vi "Accelerometer Angle.vi"(10 "angle LPF":dbl=0.02 format="%#_13g", 11 "Values":dbl[](array[numeric])) -> (3 "Numeric":dbl)   [LabVIEW 2014]
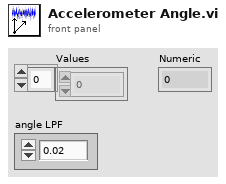
[diagram p1: front panel]
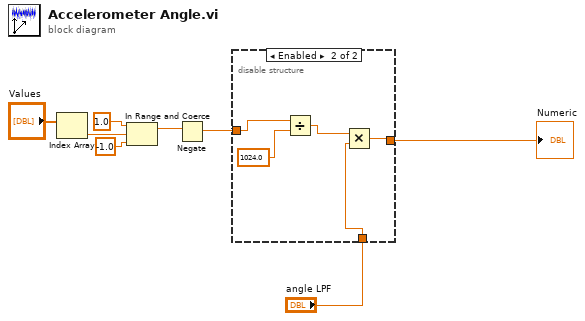
[diagram p0: block diagram]
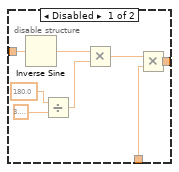
[diagram p2: hidden frame]
diagram:
  n1 = Index Array(array="Values") -> (element=w5:dbl)  [unwired: 1 in]
  n2 = In Range and Coerce(upper limit=1.0, x=w5, lower limit=-1.0) -> (coerced(x)=w8:dbl)  [unwired: 1 out]
  n3 = Negate(x=w8) -> (-x=w1:dbl)
  n4 = disable-structure shown="Enabled" {
    disable-tunnel: w1 -> [w16 w21]
    disable-tunnel: [w13 w19] -> w3
    disable-tunnel: "angle LPF" -> [w9 w18]
    frame Disabled {
      n5 = Inverse Sine(1:w16) -> (0:w14:dbl)
      n6 = Divide(x=180.0, y=3.141592653589793) -> (x/y=w12:dbl)
      n7 = Multiply(x=w14, y=w12) -> (x*y=w15:dbl)
      n8 = Multiply(x=w15, y=w9) -> (x*y=w13:dbl)
    }
    frame Enabled {
      n9 = Divide(x=w21, y=1024.0) -> (x/y=w17:dbl)
      n10 = Multiply(x=w17, y=w18) -> (x*y=w19:dbl)
    }
  }
  "Numeric" <- w3
